vi "Current_Pulse.vi"(0 "Parallel Task in":refnum<k21>, 1 "Capacity (Ah)":dbl format="%#.6g", 3 "C rate Setpoint":dbl format="%#.6g", 5 "P task error in":errorcluster, 7 "Mode (2: Charge, 3: Discharge)":i32(ring) items=["Off", "Standby", "Charge", "Discharge", "Battery"], 9 "NHR VISA in":refnum<visa-resource-name>, 11 "NHR error in":errorcluster caption="NHR error in (no error)", 12 "FilePath":path=path "C:/Users/ga11/Desktop/VI/results/3PtestCharge.lvm" caption="Filename", 13 "Wait time (s)":dbl) -> (4 "parallel task out":refnum<k21>, 6 "parallel task error out":errorcluster, 10 "VISA resource name out":refnum<visa-resource-name>, 15 "NHR error out":errorcluster)   [LabVIEW 2020]
uses:
  <vilib>/DAQmx/read.llb/DAQmx Read (Analog 1D DBL NChan 1Samp).vi
  <vilib>/DAQmx/miscellaneous.llb/DAQmx Fill In Error Info.vi
  <instrlib>/NH Research Regenerative Test Series/Public/Data/Read (Ave Current).vi
  <instrlib>/NH Research Regenerative Test Series/Public/Data/Low Level/Fetch (Ave Voltage).vi
  <instrlib>/NH Research Regenerative Test Series/Public/Data/Low Level/Fetch (Ave True Power).vi
  <instrlib>/NH Research Regenerative Test Series/NH Research Regenerative Test Series.lvlib
panel:
  out "WaitElapsed Time (s)":i32 caption="Elapsed Time (s)"
  out "Ave Current (A)":dbl
  out "Ave Voltage (V)":dbl
  out "Ave True Power (W)":dbl
  out "Status Byte Register":T1
  out "Battery1Current":dbl
  out "Battery2Current":dbl
  out "Battery3Current":dbl
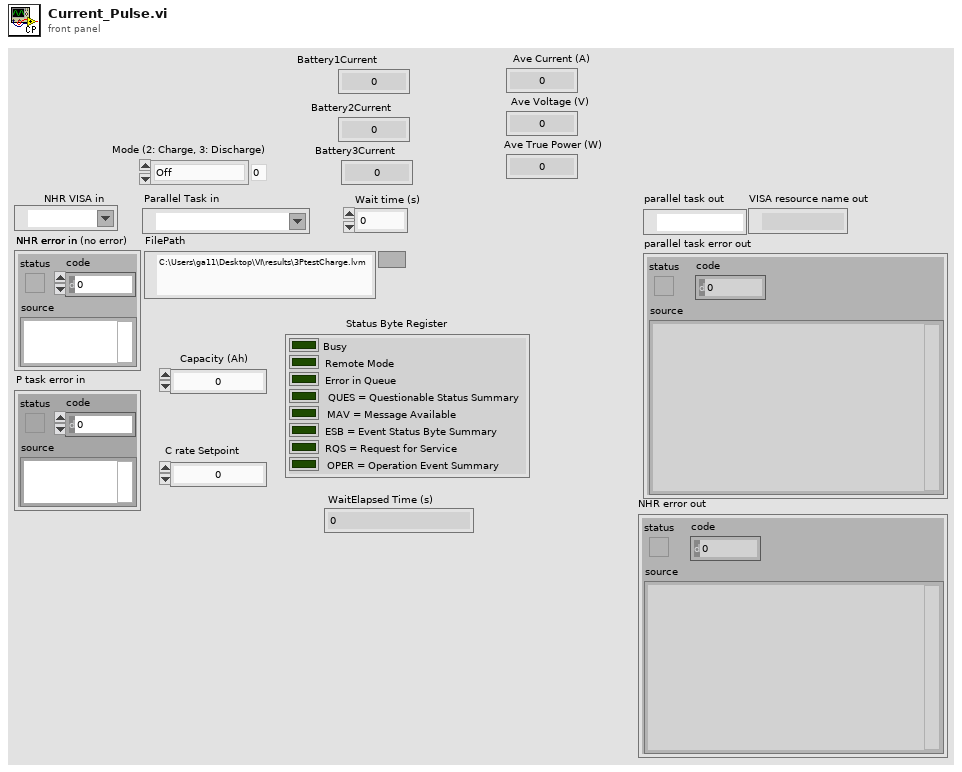
[diagram p1: front panel]
types:
  T1 = cluster{"Busy":bool, "Remote Mode":bool, "Error in Queue":bool, "QUES = Questionable Status Summary":bool, "MAV = Message Available":bool, "ESB = Event Status Byte Summary":bool, "RQS = Request for Service":bool, "OPER = Operation Event Summary":bool}
  T2 = cluster{"Voltage Enabled":bool, "Current Enabled":bool, "Power Enabled":bool, "Resistance Enabled":bool}
  T3 = cluster{"data[0]":dbl, "data[1]":dbl, "data[2]":dbl, "data[3]":dbl, "data[4]":dbl, "data[5]":dbl, "data[6]":dbl, "data[7]":dbl, "data[8]":dbl, "data[9]":dbl}
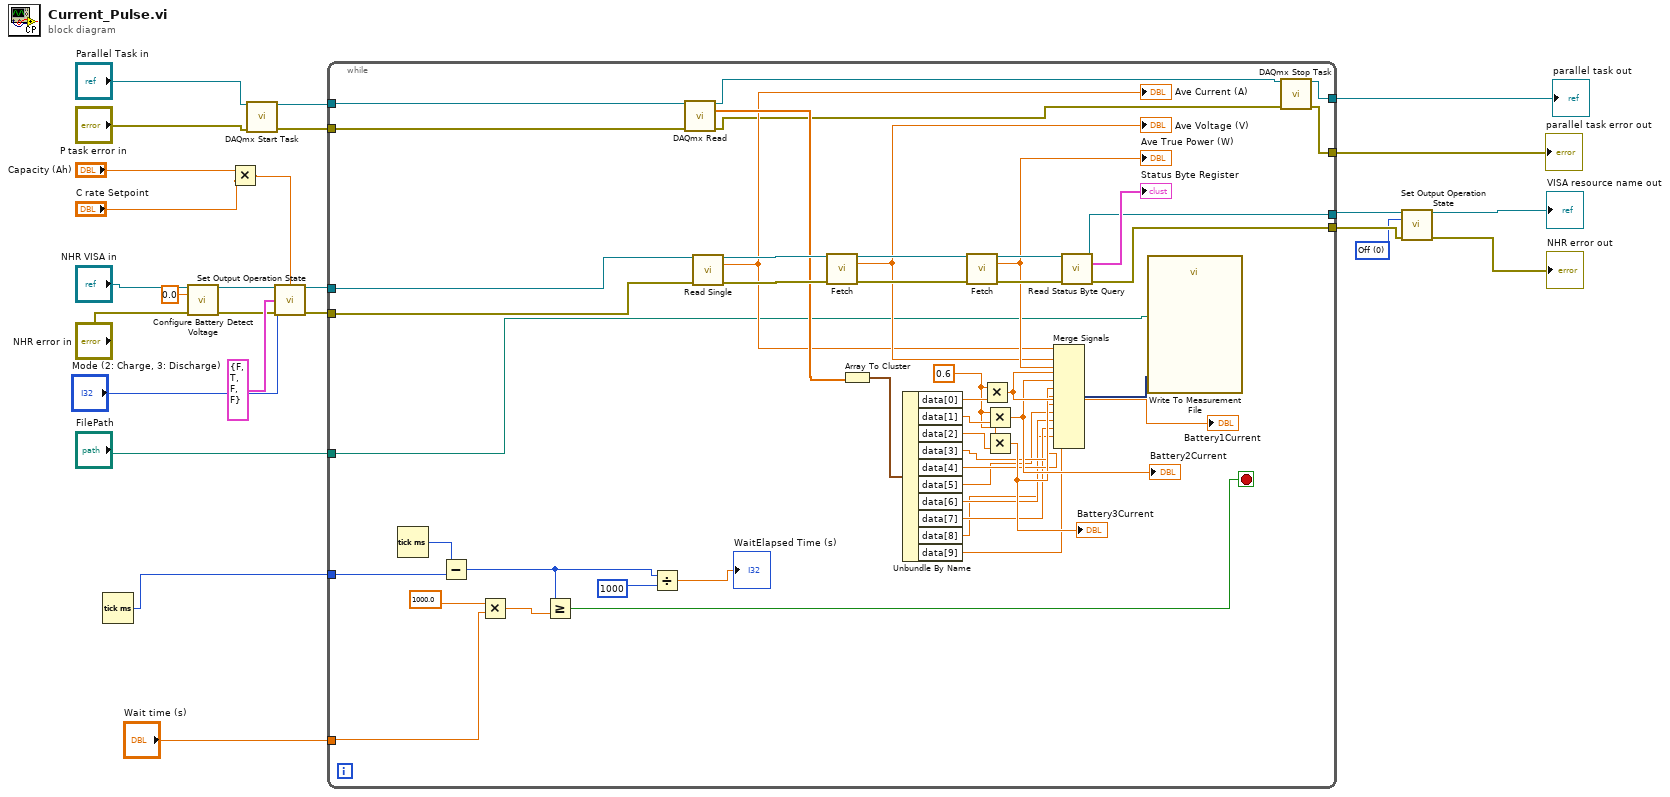
[diagram p0: block diagram]
diagram:
  w13 = 0 items=["Off", "Standby", "Charge", "Discharge", "Battery"] ("Mode (0: Off)")
  n1 = Tick Count (ms)() -> (millisecond timer value=w3:u32)
  n2 = call <instrlib>:"Configure Battery Detect Voltage.vi"("VISA resource name"="NHR VISA in", "Battery Detect Voltage (0V)"=0.0, "error in (no error)"="NHR error in") -> ("VISA resource name out"=w10:refnum<visa-resource-name>, "error out"=w9:errorcluster)  [unwired: 11 in]
  n3 = Multiply(x="Capacity (Ah)", y="C rate Setpoint") -> (x*y=w22:dbl)
  n4 = call <vilib>:"DAQmx Start Task.vi"("task/channels in"="Parallel Task in", "error in"="P task error in") -> ("task out"=w19:refnum<k21>, "error out"=w18:errorcluster)  [unwired: 12 in]
  n5 = call <vilib>:"Set Output Operation State.vi"("VISA resource name"=w10, "Current Setpoint (0 A)"=w22, "Mode (0: Off)"="Mode (2: Charge, 3: Discharge)", "Enable"=T2 {"Voltage Enabled"=FALSE, "Current Enabled"=TRUE, "Power Enabled"=FALSE, "Resistance Enabled"=FALSE}, "error in (no error)"=w9) -> ("VISA resource name out"=w26:refnum<visa-resource-name>, "error out"=w25:errorcluster)  [unwired: 9 in]
  n6 = while {
    tunnel: w26 -> [w67]
    tunnel: w25 -> [w66]
    tunnel: [w64] -> w15
    tunnel: [w63] -> w14
    tunnel: w18 -> [w42]
    tunnel: w19 -> [w41]
    tunnel: "FilePath" -> [w40]
    tunnel: [w37] -> w5
    tunnel: [w36] -> w4
    tunnel: w3 -> [w29]
    tunnel: "Wait time (s)" -> [w28]
    stop <- w27 stop-if-true
    w50 = 0.6
    n7 = Tick Count (ms)() -> (millisecond timer value=w35:u32)
    n8 = Subtract(x=w35, y=w29) -> (x-y=w32:u32)
    n9 = Multiply(x=1000.0, y=w28) -> (x*y=w33:dbl)
    n10 = Greater Or Equal?(x=w32, y=w33) -> (x >= y?=w27:bool)
    n11 = Divide(x=w32, y=1000) -> (x/y=→"WaitElapsed Time (s)":dbl)
    n12 = call-poly <vilib>:"DAQmx Read.vi"("task/channels in"=w41, "error in"=w42) -> ("task out"=w39:refnum<k21>, "data"=w61:dbl[], "error out"=w38:errorcluster)  [unwired: 11 in]
    n13 = call-poly <instrlib>:"Read Single.vi"("VISA resource name"=w67, "error in (no error)"=w66) -> ("VISA resource name out"=w72:refnum<visa-resource-name>, "Ave Current (A)"=w57:dbl, "error out"=w73:errorcluster)  [unwired: 11 in]
    "Ave Current (A)" <- w57
    n14 = call-poly <instrlib>:"Fetch.vi"("VISA resource name"=w72, "error in (no error)"=w73) -> ("VISA resource name out"=w71:refnum<visa-resource-name>, "Ave Voltage (V)"=w58:dbl, "error out"=w70:errorcluster)  [unwired: 11 in]
    "Ave Voltage (V)" <- w58
    n15 = Array To Cluster(array=w61) -> (cluster=w60:T3)
    n16 = Unbundle By Name(w60) -> ("data[0]"=w56:dbl, "data[1]"=w54:dbl, "data[2]"=w51:dbl, "data[3]"=w49:dbl, "data[4]"=w48:dbl, "data[5]"=w47:dbl, "data[6]"=w46:dbl, "data[7]"=w45:dbl, "data[8]"=w44:dbl, "data[9]"=w43:dbl)
    n17 = call-poly <instrlib>:"Fetch.vi"("VISA resource name"=w71, "error in (no error)"=w70) -> ("VISA resource name out"=w69:refnum<visa-resource-name>, "Ave True Power (W)"=w62:dbl, "error out"=w68:errorcluster)  [unwired: 11 in]
    "Ave True Power (W)" <- w62
    n18 = Multiply(x=w50, y=w56) -> (x*y=w55:dbl)
    "Battery1Current" <- w55
    n19 = Multiply(x=w50, y=w54) -> (x*y=w53:dbl)
    "Battery2Current" <- w53
    n20 = Multiply(x=w50, y=w51) -> (x*y=w52:dbl)
    "Battery3Current" <- w52
    n21 = Merge Signals "Merge Signals"(w57, w58, w62, w55, w53, w52, w49, w48, w47, w46, w45, w44, w43) -> (w59:dynamicdata)
    n22 = call <instrlib>:"Read Status Byte Query.vi"("VISA resource name"=w69, "error in (no error)"=w68) -> ("VISA resource name out"=w64:refnum<visa-resource-name>, "Status Byte Register"=→"Status Byte Register":T1, "error out"=w63:errorcluster)  [unwired: 11 in]
    n23 = call "Write To Measurement File"("Signals"=w59, "Filename"=w40) -> ()  [unwired: 15 in, 3 out]
    n24 = call <vilib>:"DAQmx Stop Task.vi"("task/channels in"=w39, "error in"=w38) -> ("task out"=w37:refnum<k21>, "error out"=w36:errorcluster)  [unwired: 12 in]
  }
  "parallel task out" <- w5
  "parallel task error out" <- w4
  n25 = call <vilib>:"Set Output Operation State.vi"("VISA resource name"=w15, "Mode (0: Off)"=w13, "error in (no error)"=w14) -> ("VISA resource name out"=→"VISA resource name out":refnum<visa-resource-name>, "error out"=→"NHR error out":errorcluster)  [unwired: 11 in]
